vi "spoofExcel.vi"(3 "Number of samples to spoof":i32=2) -> ()   [LabVIEW 2019]
uses:
  <vilib>/Utility/NIReport.llb/Report Type.ctl
  <vilib>/Utility/file.llb/Read Delimited Spreadsheet (DBL).vi
  <vilib>/addons/_office/excel.llb/Excel Easy Table (num).vi
  <vilib>/Utility/file.llb/Write Delimited Spreadsheet (DBL).vi
  <vilib>/Utility/NIReport.llb/NI_ReportGenerationCore.lvlib
  <vilib>/Utility/NIReport.llb/NI_report.lvclass
  <vilib>/addons/_office/NI_ReportGenerationToolkit.lvlib
  <vilib>/Utility/NIReport.llb/Excel/NI_Excel.lvclass
panel:
  in  "Starting Column":u32=2
  in  "Starting Row":u32=4
  in  "Output Path":path=path "C:/Users/pl9ed/Dropbox/Spring/Capstone/RPP Program/program files/working folder/test.xls"
  in  "Pattern Path - Unnecessary for random numbers":path=path "C:/Users/pl9ed/Dropbox/Spring/Capstone/data/spoof_sine_pattern.csv"
  in  "Spoof Pattern":u16(ring)=1 items=["Input", "Random"]
  in  "Write Period (ms)":u32=5000
  in  "Write Method":u16(ring) items=["Report Toolkit", "Forced filetype"]
  out "Output Values":dbl[][](array[numeric])
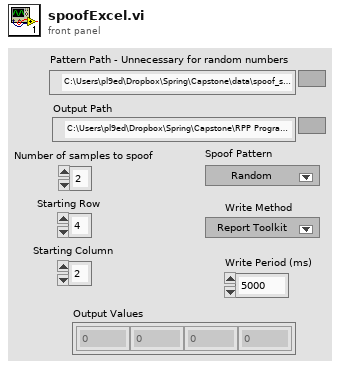
[diagram p1: front panel]
types:
  T1 = typedef "NI_ReportGenerationCore.lvlib/Report Type.ctl" = enum16{"HTML", "Word", "Excel"}
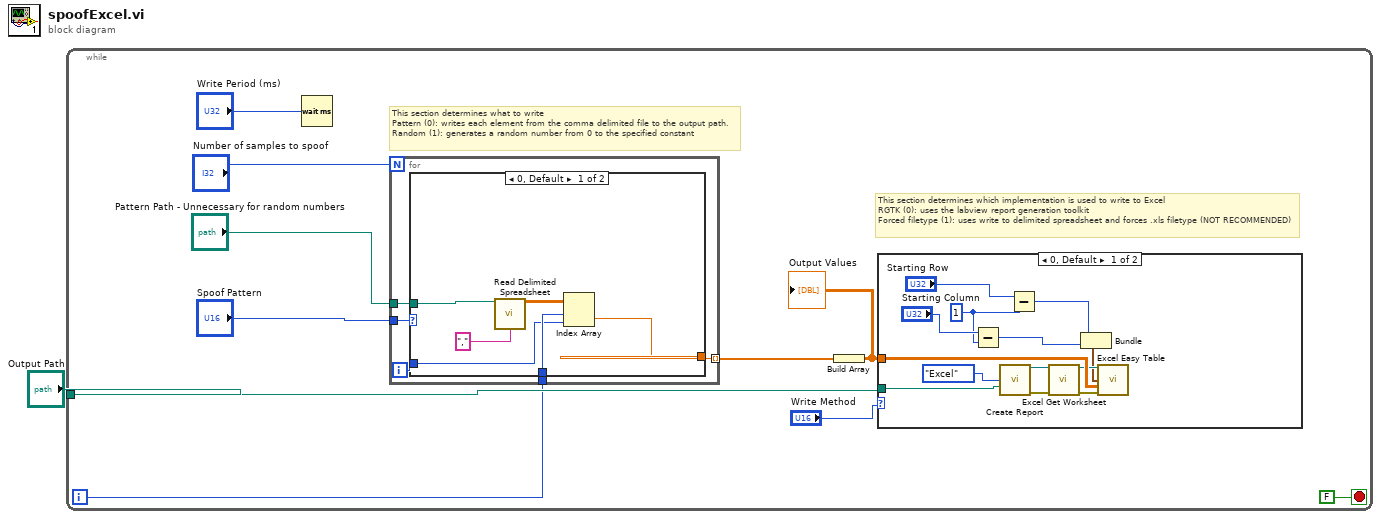
[diagram p0: block diagram]
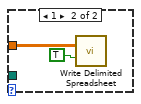
[diagram p2: hidden frame]
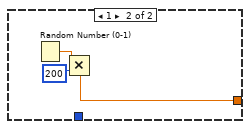
[diagram p3: hidden frame]
diagram:
  n1 = while {
    tunnel: "Output Path" -> [w6]
    i -> [w3]
    stop <- FALSE stop-if-true
    # "This section determines which implementation is used to write to Excel\nRGTK (0): uses the labview report generation toolkit \nForced filetype (1): uses write to delimited spreadsheet and forces .xls filetype (NOT RECOMMENDED)"
    # "This section determines what to write\nPattern (0): writes each element from the comma delimited file to the output path. \nRandom (1): generates a random number from 0 to the specified constant"
    n2 = Wait (ms)(milliseconds to wait="Write Period (ms)") -> ()  [unwired: 1 out]
    n3 = for {
      N: "Number of samples to spoof" -> [_]
      tunnel: [w31] -> w9 mode=indexing
      tunnel: "Spoof Pattern" -> [w30]
      tunnel: "Pattern Path - Unnecessary for random numbers" -> [w29]
      tunnel: w3 -> [w28]
      i -> [w27]
      n4 = case shown="0, Default" w30 {
        tunnel: [w33 w38] -> w31
        tunnel: w29 -> [w37 _]
        tunnel: w28 -> [w35 _]
        tunnel: w27 -> [w34 _]
        frame 0, Default {
          n5 = call-poly <vilib>:"Read Delimited Spreadsheet.vi"("file path (dialog if empty)"=w37, "delimiter (\\t)"="," ("delimiter (\\t)")) -> ("all rows"=w36:dbl[][])  [unwired: 8 in, 5 out]
          n6 = Index Array(array=w36, index (row)=w35, index (col)=w34) -> (element=w33:dbl)
        }
        frame 1 {
          n7 = Random Number (0-1)() -> (number: 0 to 1=w39:dbl)
          n8 = Multiply(x=w39, y=200) -> (x*y=w38:dbl)
        }
      }
    }
    n9 = Build Array(w9) -> (w8:dbl[][])
    "Output Values" <- w8
    n10 = case shown="0, Default" "Write Method" {
      tunnel: w8 -> [w23 w26]
      tunnel: w6 -> [w17 _]
      frame 0, Default {
        w14 = u32 1 ("y")
        n11 = Subtract(x="Starting Column", y=w14) -> (x-y=w12:u32)
        n12 = call <vilib>:"Create Report.vi"("report type"=Report_Type."Excel", "template (empty)"=w17) -> ("report out"=w22:refnum<class "NI_report.lvclass">, "error out"=w21:errorcluster)  [unwired: 12 in]
        n13 = Subtract(x="Starting Row", y=w14) -> (x-y=w13:u32)
        n14 = call <vilib>:"Excel Get Worksheet.vi"("report in"=w22, "error in (no error)"=w21) -> ("report out"=w20:refnum<class "NI_report.lvclass">, "error out"=w19:errorcluster)  [unwired: 12 in]
        n15 = Bundle(w13, w12) -> (w18:cluster{u32, u32})  [unwired: 1 in]
        n16 = call-poly <vilib>:"Excel Easy Table.vi"("report in"=w20, "start (0, 0)"=w18, "text data"=w23, "error in (no error)"=w19) -> ()  [unwired: 7 in, 5 out]
      }
      frame 1 {
        n17 = call-poly <vilib>:"Write Delimited Spreadsheet.vi"("2D data"=w26, "append to file? (new file:F)"=TRUE) -> ()  [unwired: 12 in, 2 out]
      }
    }
  }
